vi "fgv_calibration_config.vi"(6 "Non default file path?":bool, 7 "Cal config ops":T5(ring), 8 "error in (no error)":errorcluster, 10 "config file path":path, 11 "Config cluster IN":T1) -> (0 "error out":errorcluster, 2 "Config file path":path, 3 "Config cluster OUT":T1)   [LabVIEW 2020]
uses:
  Typedefs/Calibration config.ctl
  Typedefs/Objective Config.ctl
  Typedefs/Prechirper Cal Config.ctl
  Typedefs/PreChirper constants.ctl
  General Globals.vi
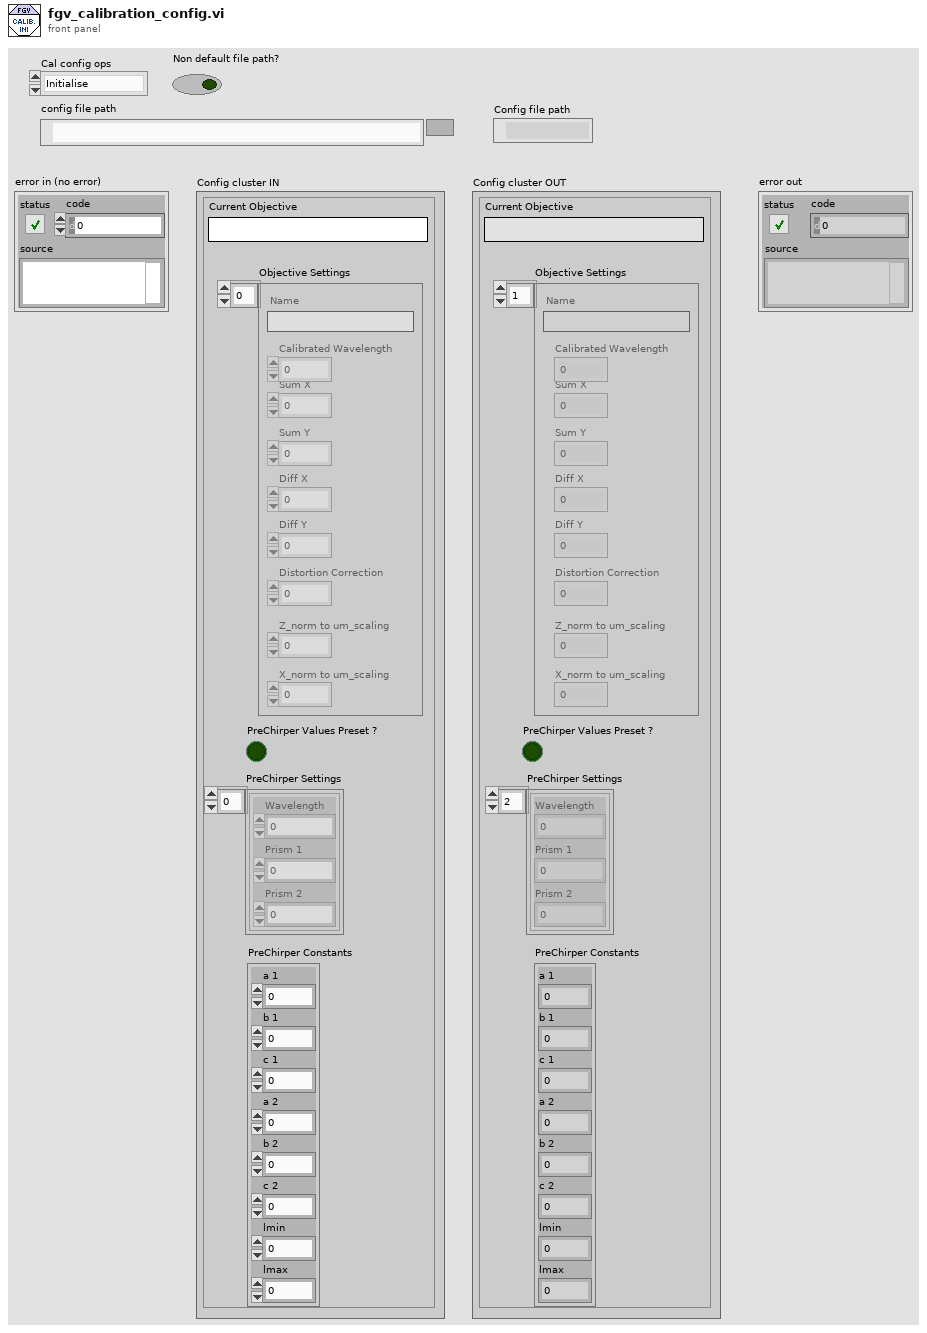
[diagram p1: front panel]
types:
  T1 = typedef "Calibration config.ctl" = cluster{"Current Objective":string, "Objective Settings":T2[], "PreChirper Values Preset ?":bool, "PreChirper Settings":T3[], "PreChirper Constants":T4}
  T2 = typedef "Objective Config.ctl" = cluster{"Name":string, "Sum X":dbl, "Sum Y":dbl, "Diff X":dbl, "Diff Y":dbl, "Distortion Correction":dbl, "Z_norm to um_scaling":dbl, "X_norm to um_scaling":dbl, "Calibrated Wavelength":dbl}
  T3 = typedef "Prechirper Cal Config.ctl" = cluster{"Wavelength":i32, "Prism 1":i32, "Prism 2":i32}
  T4 = typedef "PreChirper constants.ctl" = cluster{"a 1":i32, "b 1":i32, "c 1":i32, "a 2":i32, "b 2":i32, "c 2":i32, "lmin":i32, "lmax":i32}
  T5 = enum16{"Initialise", "Load from file", "Save to file", "Read", "Write"}
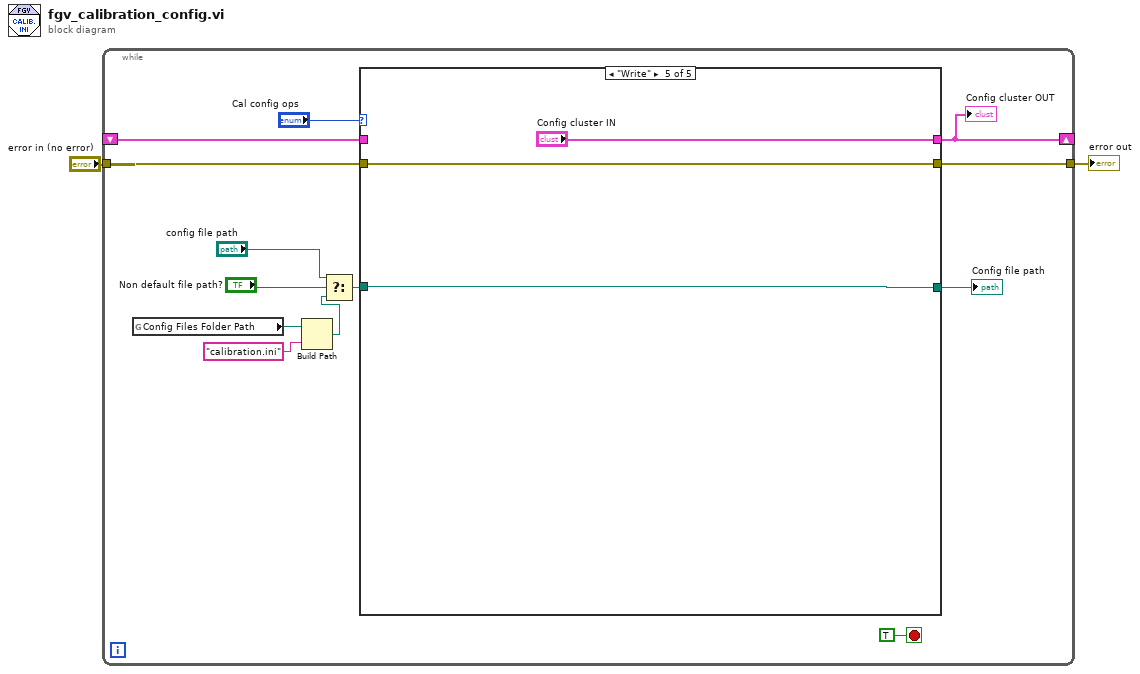
[diagram p0: block diagram]
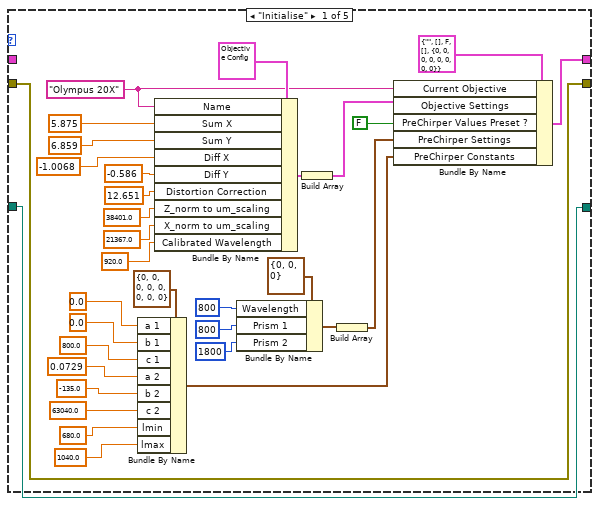
[diagram p2: hidden frame]
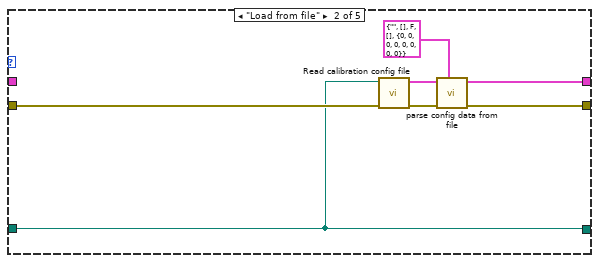
[diagram p3: hidden frame]
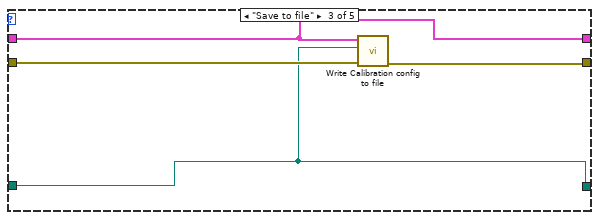
[diagram p4: hidden frame]
diagram:
  n1 = while {
    tunnel: "error in (no error)" -> [w13]
    shift-right: [w10] -> _
    shift-left: _ -> [w12]
    tunnel: [w11] -> w1
    stop <- TRUE stop-if-true
    n2 = global read "General Globals.vi" "Config Files Folder Path"() -> (w8:path)
    n3 = Build Path(base path=w8, name or relative path="calibration.ini") -> (appended path=w4:path)
    n4 = Select(t="config file path", s="Non default file path?", f=w4) -> (s? t:f=w3:path)
    n5 = case shown="\"Write\"" "Cal config ops" {
      tunnel: w13 -> [w29 w53 w59 w62 w64]
      tunnel: [w29 w52 w58 w62 w64] -> w11
      tunnel: [w30 w51 w57 w61 "Config cluster IN"] -> w10
      tunnel: w12 -> [_ _ w57 w61 _]
      tunnel: [w16 w50 w56 w60 w63] -> w9
      tunnel: w3 -> [w16 w50 w56 w60 w63]
      frame "Initialise" {
        w46 = "Olympus 20X" ("Current Objective")
        n6 = Bundle By Name(cluster=T4 {"a 1"=0, "b 1"=0, "c 1"=0, "a 2"=0, "b 2"=0, "c 2"=0, "lmin"=0, "lmax"=0} ("Prechirper Constants"), "a 1"=0.0, "b 1"=0.0, "c 1"=800.0, "a 2"=0.0729, "b 2"=-135.0, "c 2"=63040.0, "lmin"=680.0, "lmax"=1040.0) -> (w19:T4)
        n7 = Bundle By Name(cluster=T2 {"Name"="", "Sum X"=0.0, "Sum Y"=0.0, "Diff X"=0.0, "Diff Y"=0.0, "Distortion Correction"=0.0, "Z_norm to um_scaling"=0.0, "X_norm to um_scaling"=0.0, "Calibrated Wavelength"=0.0} ("Objective HW Settings"), "Name"=w46, "Sum X"=5.875, "Sum Y"=6.859, "Diff X"=-1.0068 ("Sum Y"), "Diff Y"=-0.586 ("Sum Y"), "Distortion Correction"=12.651 ("Sum Y"), "Z_norm to um_scaling"=38401.0 ("Sum Y"), "X_norm to um_scaling"=21367.0 ("Sum Y"), "Calibrated Wavelength"=920.0) -> (w37:T2)
        n8 = Bundle By Name(cluster=T3 {"Wavelength"=0, "Prism 1"=0, "Prism 2"=0} ("Prechirper Config"), "Wavelength"=800, "Prism 1"=800, "Prism 2"=1800) -> (w33:T3)
        n9 = Build Array(w37) -> (w36:T2[])
        n10 = Build Array(w33) -> (w18:T3[])
        n11 = Bundle By Name(cluster=T1 {"Current Objective"="", "Objective Settings"=[], "PreChirper Values Preset ?"=FALSE, "PreChirper Settings"=[], "PreChirper Constants"={"a 1"=0, "b 1"=0, "c 1"=0, "a 2"=0, "b 2"=0, "c 2"=0, "lmin"=0, "lmax"=0}} ("Config cluster IN"), "Current Objective"=w46, "Objective Settings"=w36, "PreChirper Values Preset ?"=FALSE, "PreChirper Settings"=w18, "PreChirper Constants"=w19) -> (w30:T1)
      }
      frame "Load from file" {
        n12 = call "Read calibration config file.vi"("error in (no error)"=w53, "configuration file path"=w50) -> ("error out"=w54:errorcluster, "Array"=w55:cluster{"String":string, string[]}[])  [unwired: 8 in]
        n13 = call "parse config data from file.vi"("Calibration Config"=T1 {"Current Objective"="", "Objective Settings"=[], "PreChirper Values Preset ?"=FALSE, "PreChirper Settings"=[], "PreChirper Constants"={"a 1"=0, "b 1"=0, "c 1"=0, "a 2"=0, "b 2"=0, "c 2"=0, "lmin"=0, "lmax"=0}}, "Error in"=w54, "Array"=w55) -> ("Error out"=w52:errorcluster, "Config cluster"=w51:T1)  [unwired: 7 in]
      }
      frame "Save to file" {
        n14 = call "Write Calibration config to file.vi"("error in (no error)"=w59, "configuration file path"=w56, "Calibration config."=w57) -> ("error out"=w58:errorcluster)  [unwired: 8 in]
      }
      frame "Read", Default {
      }
      frame "Write" {
      }
    }
    "Config cluster OUT" <- w10
    "Config file path" <- w9
  }
  "error out" <- w1
